vi "Error Process.vi"(8 "error in (no error)":errorcluster, 11 "View Model":T1) -> (0 "error out":errorcluster, 3 "View Model":T1)   [LabVIEW 2017]
uses:
  View Model/Controls/View Model.ctl
  Configuration Database/Controls/Config Model.ctl
  Configuration Database/Controls/Congif Data.ctl
  Configuration Database/Controls/Config Commands.ctl
  View Model/Controls/Shared Model.ctl
  Controls/Error Model.ctl
  Controls/Error Data.ctl
  Controls/Error Type.ctl
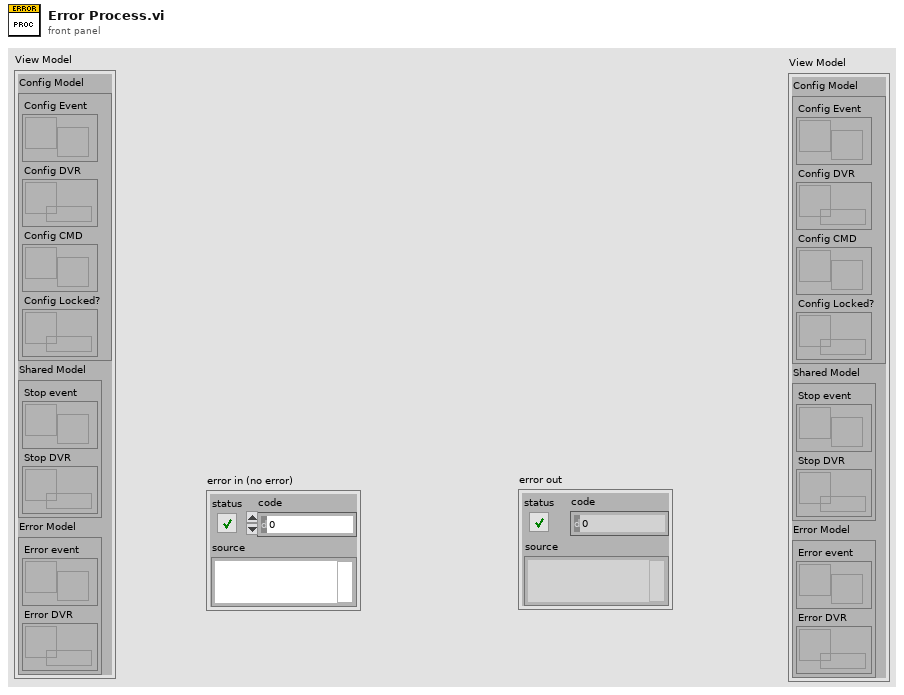
[diagram p1: front panel]
types:
  T1 = typedef "View Model.ctl" = cluster{"Config Model":T2, "Shared Model":T3, "Error Model":T4}
  T2 = typedef "Config Model.ctl" = cluster{"Config Event":refnum<user-event>, "Config DVR":refnum<data-value>, "Config CMD":refnum<user-event>, "Config Locked?":refnum<data-value>}
  T3 = typedef "Shared Model.ctl" = cluster{"Stop event":refnum<user-event>, "Stop DVR":refnum<data-value>}
  T4 = typedef "Error Model.ctl" = cluster{"Error event":refnum<user-event>, "Error DVR":refnum<data-value>}
  T5 = typedef "Error Data.ctl" = cluster{"Error Type":T6, "Error cluster":errorcluster, "Other Data":variant}
  T6 = typedef "Error Type.ctl" = enum16{"Minor Error", "Wash Cycle Error", "System Error", "Other Error"}
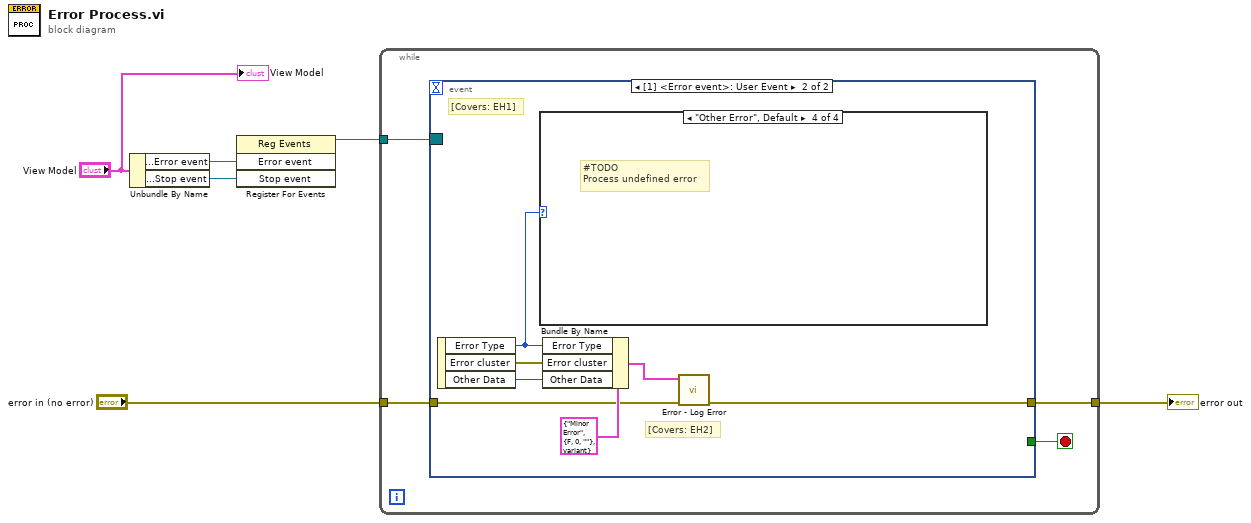
[diagram p0: block diagram]
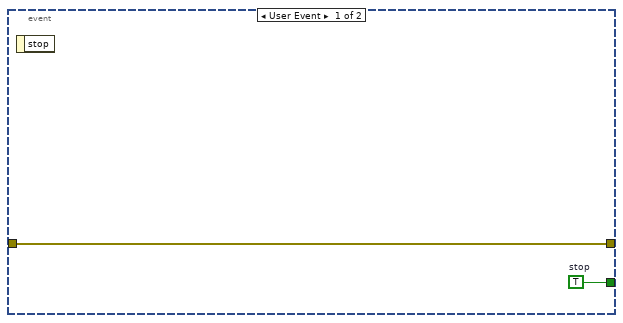
[diagram p2: hidden frame]
diagram:
  n1 = Unbundle By Name("View Model") -> ("Error Model.Error event"=w6:refnum<user-event>, "Shared Model.Stop event"=w5:refnum<user-event>)
  n2 = register-events(w6, w5) -> (reference out=w4:refnum<event-registration>)  [unwired: 2 in, 1 out]
  n3 = while {
    tunnel: w4 -> [w10]
    tunnel: "error in (no error)" -> [w8]
    tunnel: [w7] -> w1
    stop <- w9 stop-if-true
    n4 = event shown="[1] <Error event>: User Event" {
      selector: w10 -> [_ _]
      dyn-events: _ -> [_ _]
      timeout: _ -> [_ _]
      tunnel: [w12 _] -> w9
      tunnel: w8 -> [w11 w15]
      tunnel: [w11 w14] -> w7
      event User Event {
        w12 = TRUE  # stop
        n5 = event-data() -> ()  [unwired: 1 in, 1 out]
      }
      event User Event {
        # "[Covers: EH1]"
        # "[Covers: EH2]"
        n6 = event-data() -> ("Error Type"=w13:T6, "Error cluster"=w17:errorcluster, "Other Data"=w18:variant)  [unwired: 1 in]
        n7 = case shown="\"Other Error\", Default" w13 {
          frame "Minor Error" {
            # "[Covers: EH1A]"
            # "#TODO\nThis error should be invisible to the user\nContinues any operations without interruption"
          }
          frame "Wash Cycle Error" {
            # "[Covers: EH1B2]"
            # "[Covers: EH1B1]"
            # "[Covers: EH1B]"
            # "#TODO\n- Enter the Wash Abort/Terminate state\n- Displays an Error Dialog with message for user\n to move car to the Exit position\n- Prepare controller to run a new wash cycle"
          }
          frame "System Error" {
            # "[Covers: EH1C3]"
            # "[Covers: EH1C2]"
            # "[Covers: EH1C1]"
            # "[Covers: EH1C]"
            # "#TODO\nLocks out the system and cause the system to enter the\nWash Abort/Terminate state\n- Causes a shutdown of all consoles and hardware\n- Displays an Error Dialog with message for user to move car to the Exit position.\n- Terminate the application."
          }
          frame "Other Error", Default {
            # "#TODO\nProcess undefined error"
          }
        }
        n8 = Bundle By Name(cluster=T5 {"Error Type"=enum."Minor Error", "Error cluster"={"status"=FALSE, "code"=0, "source"=""}, "Other Data"=variant} ("Error Data"), "Error Type"=w13, "Error cluster"=w17, "Other Data"=w18) -> (w16:T5)
        n9 = call "Error - Log Error.vi"("error in (no error)"=w15, "Error Data"=w16) -> ("error out"=w14:errorcluster)  [unwired: 9 in]
      }
    }
  }
  "error out" <- w1
  "View Model" <- "View Model"
